vi "TX_POWER.vi"() -> ()   [LabVIEW 2015]
uses:
  Global_Instr.vi
  Global_GET_INSTRSTATE.vi
  <instrlib>/Rohde&Schwarz Spectrum Analyzer/Rohde&Schwarz Spectrum Analyzer.lvlib
panel:
  in  "fs":dbl=125000000.0
  in  "fnco":dbl=190000000.0
  out "Bx":dbl[](array[numeric]) caption="X" format="%^.3e"
  out "By":dbl[](array[numeric]) caption="Amplitude" format="%^.3e"
  out "B_posB":dbl caption="Marker Position" format="%^.3e"
  out "B_peak":dbl caption="Marker Amplitude" format="%^.3e"
  out "B_next_pos":dbl caption="Marker Position" format="%^.3e"
  out "B_peak_next":dbl caption="Marker Amplitude" format="%^.3e"
  out "A_peak_next":dbl caption="Marker Amplitude" format="%^.3e"
  out "A_next_pos":dbl caption="Marker Position" format="%^.3e"
  out "A_peak":dbl caption="Marker Amplitude" format="%^.3e"
  out "A_pos":dbl caption="Marker Position" format="%^.3e"
  out "Ay":dbl[](array[numeric]) caption="Amplitude" format="%^.3e"
  out "Ax":dbl[](array[numeric]) caption="X" format="%^.3e"
  in  "VISA resource name 2":refnum<visa-resource-name>="COM3"
  out "Freq_Tab":u32[](array[numeric])
  in  "Insert Point":u32
  in  "EABLE Insert":bool
  in  "Value":u32=10 caption="Point Num"
  in  "cnt/setp":enum16{"SETP", "COUNT"}(ring)=enum."COUNT"
  in  "freq_max(Mhz)":u32=2123
  in  "freq_min(Mhz)":u32=2000
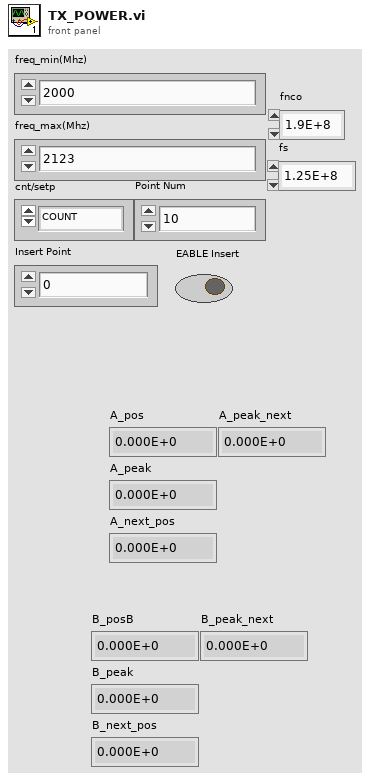
[diagram p1: front panel]
types:
  T1 = cluster{"Serial_state":bool, "key#4_state":bool, "key#6_state":bool, "spec1_state":bool, "spec2_state":bool, "sma100_state":bool}
  T2 = cluster{"O_Serial":refnum<visa-resource-name>, "O_KEY#6":refnum<visa-resource-name>, "O_key#4":refnum<visa-resource-name>, "O_R&S_SMA100":refnum<visa-resource-name>, "O_R&S Spec1":refnum<visa-resource-name>, "O_R&S Spec2":refnum<visa-resource-name>}
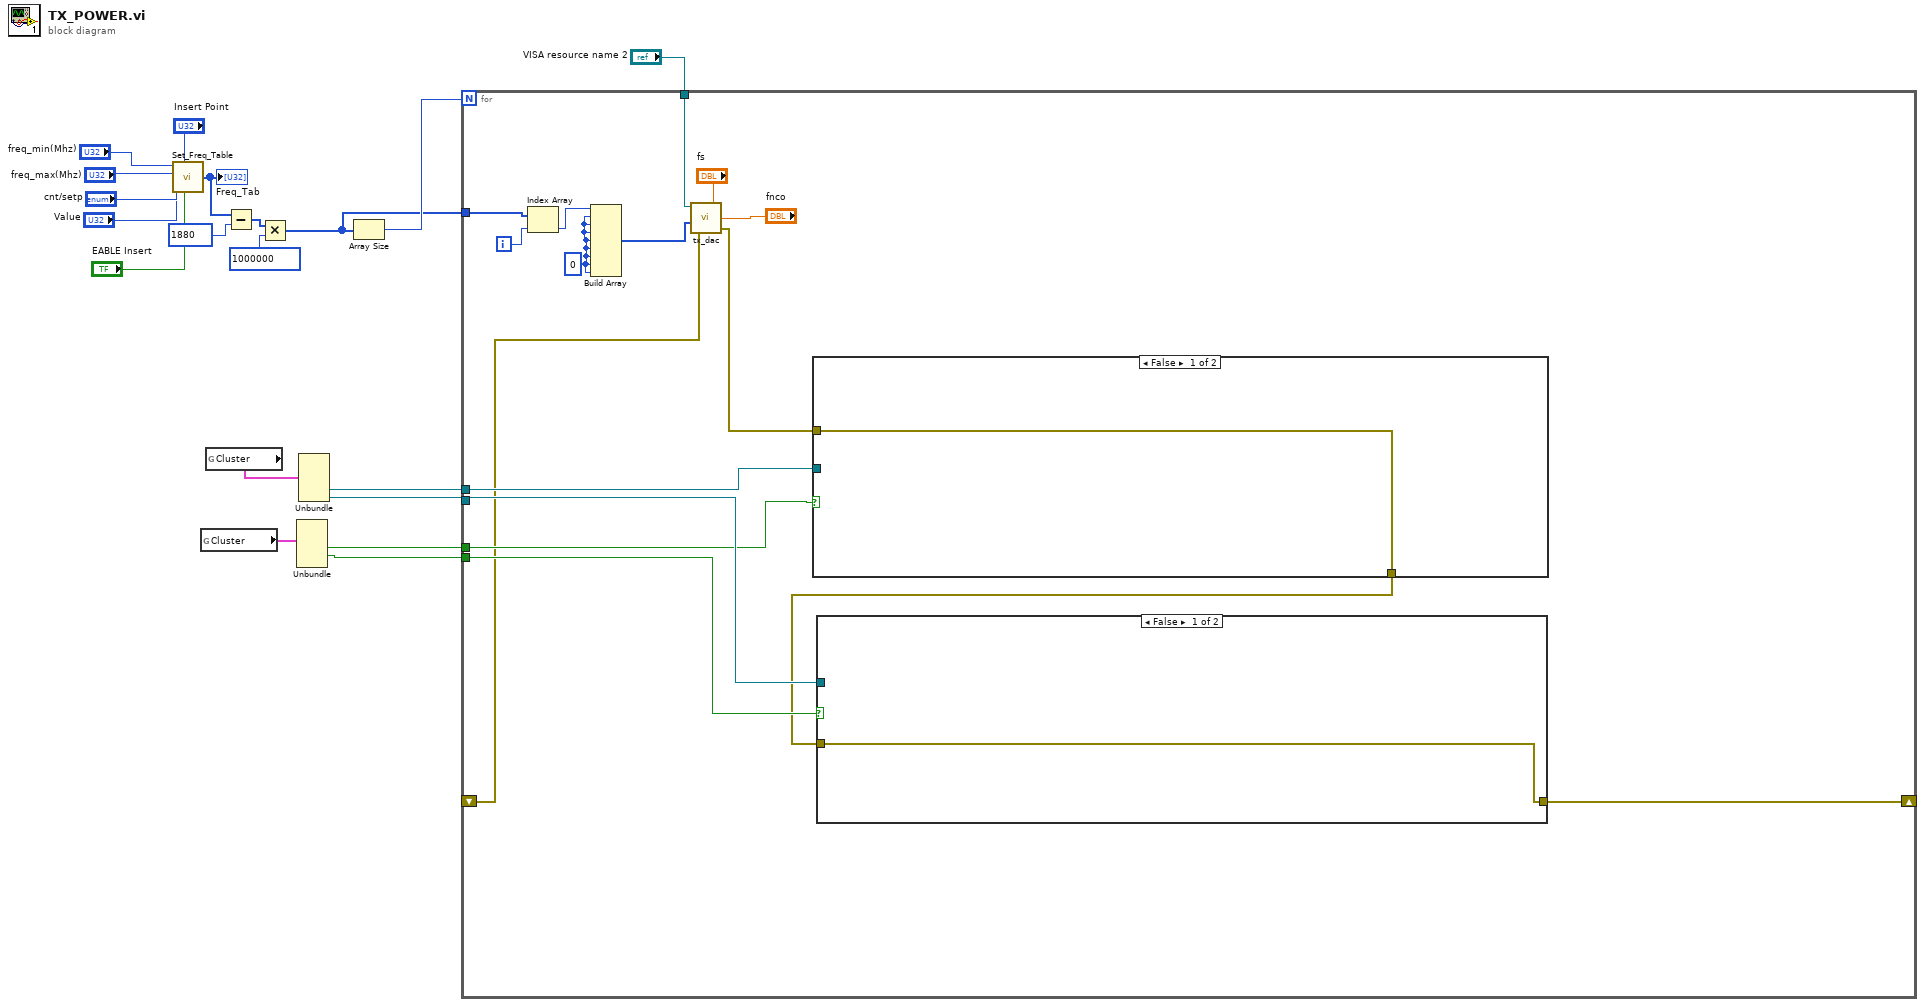
[diagram p0: block diagram]
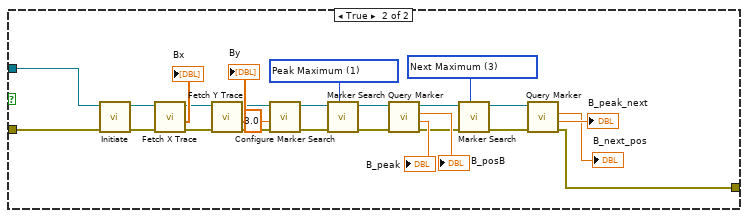
[diagram p2: hidden frame]
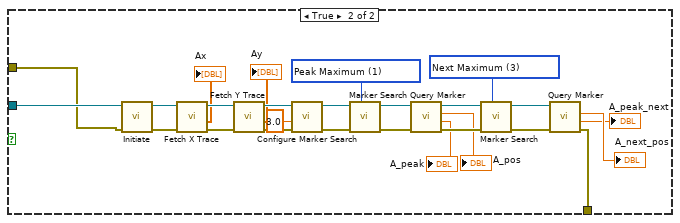
[diagram p3: hidden frame]
diagram:
  n1 = call "Set_Freq_Table.vi"("EABLE Insert"="EABLE Insert", "Insert Point"="Insert Point", "Value"="Value", "cnt/setp"="cnt/setp", "freq_max(Mhz)"="freq_max(Mhz)", "freq_min(Mhz)"="freq_min(Mhz)") -> ("Freq_Tab"=w13:u32[])
  "Freq_Tab" <- w13
  n2 = global read "Global_GET_INSTRSTATE.vi" "Cluster"() -> (w4:T1)
  n3 = global read "Global_Instr.vi" "Cluster"() -> (w6:T2)
  n4 = Subtract(x=w13, y=1880) -> (x-y=w11:u32[])
  n5 = Multiply(x=w11, y=1000000) -> (x*y=w8:u32[])
  n6 = Unbundle(w4) -> ("spec1_state"=w2:bool, "spec2_state"=w1:bool)  [unwired: 4 out]
  n7 = Unbundle(w6) -> ("O_R&S Spec1"=w5:refnum<visa-resource-name>, "O_R&S Spec2"=w3:refnum<visa-resource-name>)  [unwired: 4 out]
  n8 = Array Size(array=w8) -> (size(s)=w9:i32)
  n9 = for {
    N: w9 -> [_]
    tunnel: w8 -> [w34]
    tunnel: "VISA resource name 2" -> [w33]
    tunnel: w5 -> [w29]
    tunnel: w3 -> [w28]
    tunnel: w2 -> [w27]
    tunnel: w1 -> [w26]
    shift-right: [w21] -> _
    shift-left: _ -> [w20]
    i -> [w35]
    w30 = u32 0 ("element")
    n10 = Index Array(array=w34, index=w35) -> (element=w31:u32)
    n11 = Build Array(w31, w30, w30, w30, w30, w30, w30, w30, w30) -> (w32:u32[])
    n12 = call "tx_dac.vi"("fnco"="fnco", "fs"="fs", "error in (no error)"=w20, "fin"=w32, "VISA resource name 2"=w33) -> ("error out"=w23:errorcluster)  [unwired: 1 in]
    n13 = case shown="False" w27 {
      tunnel: w29 -> [_ w66]
      tunnel: w23 -> [w63 w65]
      tunnel: [w63 w64] -> w22
      frame False {
      }
      frame True {
        w71 = 3 items=["Peak Maximum"=1, "Peak Minimum"=2, "Next Maximum"=3, "Left Maximum"=4, "Right Maximum"=5, "Next Minimum"=6, "Left Minimum"=7, "Right Minimum"=8] ("Marker Search (Peak Maximum)")
        w72 = 1 items=["Peak Maximum"=1, "Peak Minimum"=2, "Next Maximum"=3, "Left Maximum"=4, "Right Maximum"=5, "Next Minimum"=6, "Left Minimum"=7, "Right Minimum"=8] ("Marker Search (Peak Maximum)")
        n14 = call <instrlib>:"Initiate.vi"("error in (no error)"=w65, "VISA resource name"=w66) -> ("error out"=w89:errorcluster, "VISA resource name out"=w88:refnum<visa-resource-name>)  [unwired: 8 in]
        n15 = call <instrlib>:"Fetch X Trace.vi"("error in (no error)"=w89, "VISA resource name"=w88) -> ("error out"=w87:errorcluster, "X"=→"Ax":dbl[], "VISA resource name out"=w86:refnum<visa-resource-name>)  [unwired: 7 in]
        n16 = call <instrlib>:"Fetch Y Trace.vi"("error in (no error)"=w87, "VISA resource name"=w86) -> ("error out"=w85:errorcluster, "Amplitude"=→"Ay":dbl[], "VISA resource name out"=w84:refnum<visa-resource-name>)  [unwired: 7 in]
        n17 = call <instrlib>:"Configure Marker Search.vi"("error in (no error)"=w85, "Peak Excursion (6.0)"=3.0, "VISA resource name"=w84) -> ("error out"=w83:errorcluster, "VISA resource name out"=w82:refnum<visa-resource-name>)  [unwired: 7 in]
        n18 = call <instrlib>:"Marker Search.vi"("Marker Search (Peak Maximum)"=w72, "error in (no error)"=w83, "VISA resource name"=w82) -> ("error out"=w81:errorcluster, "VISA resource name out"=w80:refnum<visa-resource-name>)  [unwired: 7 in]
        n19 = call <instrlib>:"Query Marker.vi"("error in (no error)"=w81, "VISA resource name"=w80) -> ("error out"=w79:errorcluster, "Marker Amplitude"=→"A_peak":dbl, "Marker Position"=→"A_pos":dbl, "VISA resource name out"=w78:refnum<visa-resource-name>)  [unwired: 6 in]
        n20 = call <instrlib>:"Marker Search.vi"("Marker Search (Peak Maximum)"=w71, "error in (no error)"=w79, "VISA resource name"=w78) -> ("error out"=w77:errorcluster, "VISA resource name out"=w76:refnum<visa-resource-name>)  [unwired: 7 in]
        n21 = call <instrlib>:"Query Marker.vi"("error in (no error)"=w77, "VISA resource name"=w76) -> ("error out"=w64:errorcluster, "Marker Amplitude"=→"A_peak_next":dbl, "Marker Position"=→"A_next_pos":dbl)  [unwired: 6 in, 1 out]
      }
    }
    n22 = case shown="False" w26 {
      tunnel: w28 -> [_ w39]
      tunnel: w22 -> [w36 w38]
      tunnel: [w36 w37] -> w21
      frame False {
      }
      frame True {
        w58 = 3 items=["Peak Maximum"=1, "Peak Minimum"=2, "Next Maximum"=3, "Left Maximum"=4, "Right Maximum"=5, "Next Minimum"=6, "Left Minimum"=7, "Right Minimum"=8] ("Marker Search (Peak Maximum)")
        w57 = 1 items=["Peak Maximum"=1, "Peak Minimum"=2, "Next Maximum"=3, "Left Maximum"=4, "Right Maximum"=5, "Next Minimum"=6, "Left Minimum"=7, "Right Minimum"=8] ("Marker Search (Peak Maximum)")
        n23 = call <instrlib>:"Initiate.vi"("error in (no error)"=w38, "VISA resource name"=w39) -> ("error out"=w40:errorcluster, "VISA resource name out"=w41:refnum<visa-resource-name>)  [unwired: 8 in]
        n24 = call <instrlib>:"Fetch X Trace.vi"("error in (no error)"=w40, "VISA resource name"=w41) -> ("error out"=w42:errorcluster, "X"=→"Bx":dbl[], "VISA resource name out"=w43:refnum<visa-resource-name>)  [unwired: 7 in]
        n25 = call <instrlib>:"Fetch Y Trace.vi"("error in (no error)"=w42, "VISA resource name"=w43) -> ("error out"=w44:errorcluster, "Amplitude"=→"By":dbl[], "VISA resource name out"=w45:refnum<visa-resource-name>)  [unwired: 7 in]
        n26 = call <instrlib>:"Configure Marker Search.vi"("error in (no error)"=w44, "Peak Excursion (6.0)"=3.0, "VISA resource name"=w45) -> ("error out"=w46:errorcluster, "VISA resource name out"=w47:refnum<visa-resource-name>)  [unwired: 7 in]
        n27 = call <instrlib>:"Marker Search.vi"("Marker Search (Peak Maximum)"=w57, "error in (no error)"=w46, "VISA resource name"=w47) -> ("error out"=w48:errorcluster, "VISA resource name out"=w49:refnum<visa-resource-name>)  [unwired: 7 in]
        n28 = call <instrlib>:"Query Marker.vi"("error in (no error)"=w48, "VISA resource name"=w49) -> ("error out"=w50:errorcluster, "Marker Amplitude"=→"B_peak":dbl, "Marker Position"=→"B_posB":dbl, "VISA resource name out"=w51:refnum<visa-resource-name>)  [unwired: 6 in]
        n29 = call <instrlib>:"Marker Search.vi"("Marker Search (Peak Maximum)"=w58, "error in (no error)"=w50, "VISA resource name"=w51) -> ("error out"=w52:errorcluster, "VISA resource name out"=w53:refnum<visa-resource-name>)  [unwired: 7 in]
        n30 = call <instrlib>:"Query Marker.vi"("error in (no error)"=w52, "VISA resource name"=w53) -> ("error out"=w37:errorcluster, "Marker Amplitude"=→"B_peak_next":dbl, "Marker Position"=→"B_next_pos":dbl)  [unwired: 6 in, 1 out]
      }
    }
  }
